vi "Save Image As Binary File LV2012 NIVerified.vi"() -> ()   [LabVIEW 2012]
doc: "This VI demonstrates how to write an image as binary file."
panel:
  out "Pixels saved":i32
  out "Picture height":i32
  out "Picture width":i32
  in  "Picture to save":picture
  # "Overview: Demonstrates how to write an image as binary file. \nRequirements: LabVIEW Base Development System 2012 (or compatible)\nInstructions: \n1. Run the VI to create file called BinaryImage.bin in the folder of the VI.\n2. Open and run Load Image From Binary File.vi"
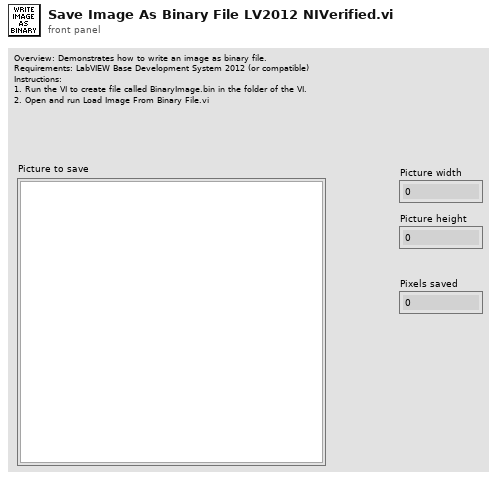
[diagram p1: front panel]
types:
  T1 = enum16{"big-endian, network order", "native, host order", "little-endian"}
  T2 = enum16{"open", "replace", "create", "open or create", "replace or create", "replace or create with confirmation"}
  T3 = typedef "imagedata.ctl" = cluster{"image type":i32, "image depth":i32, "image":u8[], "mask":u8[], "colors":u32[], "Rectangle":cluster{"left":i16, "top":i16, "right":i16, "bottom":i16}}
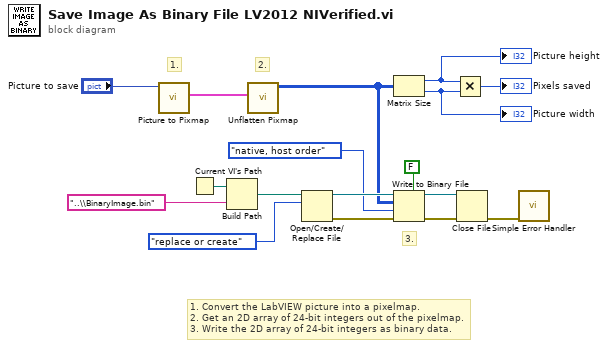
[diagram p0: block diagram]
diagram:
  # "1. Convert the LabVIEW picture into a pixelmap.\n2. Get an 2D array of 24-bit integers out of the pixelmap. \n3. Write the 2D array of 24-bit integers as binary data."
  # "3."
  # "2."
  # "1."
  n1 = call <vilib>:"Picture to Pixmap.vi"("picture"="Picture to save") -> ("image data"=w7:T3)  [unwired: 9 in, 1 out]
  n2 = Current VI's Path() -> (path=w11:path)
  n3 = Build Path(base path=w11, name or relative path="..\\BinaryImage.bin") -> (appended path=w10:path)
  n4 = call <vilib>:"Unflatten Pixmap.vi"("image data"=w7) -> ("24-bit pixmap"=w2:u32[][])  [unwired: 4 in, 6 out]
  n5 = Open/Create/Replace File(file path (use dialog)=w10, operation (0:open)=T2."replace or create") -> (refnum out=w14:refnum<file>, error out=w17:errorcluster)  [unwired: 4 in, 1 out]
  n6 = Matrix Size(0:w2) -> (1:w4:i32, 2:w3:i32)
  "Picture width" <- w3
  "Picture height" <- w4
  n7 = Write to Binary File(file (use dialog)=w14, data=w2, error in=w17, 5:FALSE ("prepend array or string size? (T)"), 9:T1."native, host order" ("byte order (0:big-endian, network order)")) -> (refnum out=w15:refnum<file>, error out=w16:errorcluster)  [unwired: 1 in, 1 out]
  n8 = Multiply(x=w4, y=w3) -> (x*y=→"Pixels saved":i32)
  n9 = Close File(refnum=w15, error in=w16) -> (error out=w8:errorcluster)  [unwired: 1 out]
  n10 = call <vilib>:"Simple Error Handler.vi"("error in (no error)"=w8) -> ()  [unwired: 4 in, 5 out]
